vi "Handle mouse enter.vi"(8 "error in (no error)":errorcluster, 11 "DatagridElement in":refnum<class "DatagridElement.lvclass">) -> (0 "error out":errorcluster, 2 "Active cursor":u16, 3 "DatagridElement out":refnum<class "DatagridElement.lvclass">)   [LabVIEW 2020, in "D Datagrid Library.lvlib" / "DatagridElement.lvclass"]
doc: "Sets the mouseover cursor for this element. Override this VI for each child that needs a custom (non-automatic) cursor."
uses:
  DatagridElement.lvclass
  DatagridElement.lvclass/DatagridElement.ctl
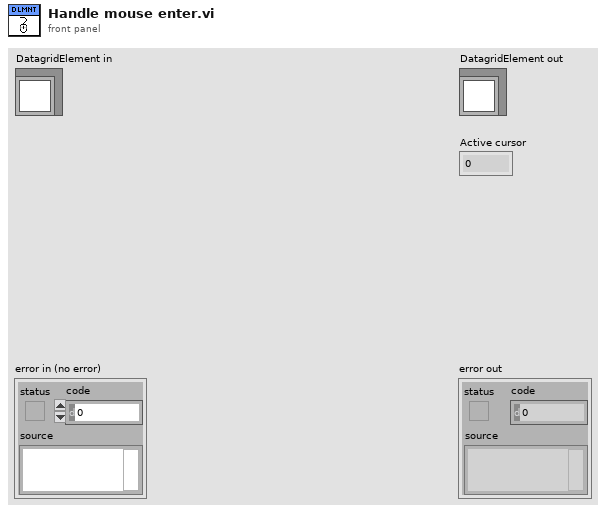
[diagram p1: front panel]
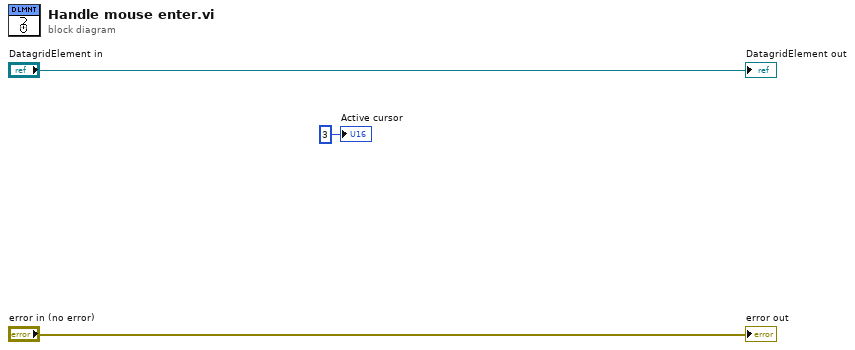
[diagram p0: block diagram]
diagram:
  "error out" <- "error in (no error)"
  "DatagridElement out" <- "DatagridElement in"
  "Active cursor" <- u16 3 ("icon")
